vi "NI-DAQmxUpdate.vi"() -> (0 "error out":errorcluster)   [LabVIEW 2022 SP3]
uses:
  Sub_vis/Upload Data.ctl
  <vilib>/DAQmx/read.llb/DAQmx Read (Analog 2D DBL NChan NSamp).vi
  Globals/Meas_global.vi
  <vilib>/DAQmx/create/channels.llb/DAQmx Create Channel (AI-Voltage-Basic).vi
  PWA/PWAtasksGLOBAL.vi
  <vilib>/DAQmx/configure/timing.llb/DAQmx Timing (Sample Clock).vi
  <vilib>/DAQmx/miscellaneous.llb/DAQmx Fill In Error Info.vi
  <resource>/objmgr/daqmx.rc
  5b8cb71c-e545-4ba2-a204-efceee465973.vi
panel:
  out "bufferSizeAssigned":u32
  out "totalPlannedSamples":i32
  out "Array":string[](array[string])
  out "Requested No of blocks":i32
  out "Current Block No":i32
  out "FsReq":dbl
  out "FsRead":dbl format="%#_11g"
  out "input terminal configuration":i32(ring)=10106 items=["default"=-1, "RSE"=10083, "NRSE"=10078, "Differential"=10106, "Pseudodifferential"=12529]
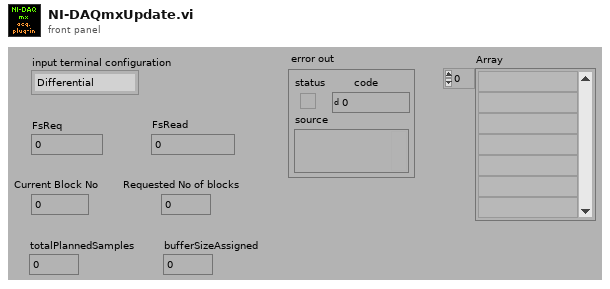
[diagram p1: front panel]
types:
  T1 = typedef "Analysis_info_cluster.ctl" = cluster{"Colour":u32, "Inst type":T2, "Inst name":string, "Symbol":string, "Code name":string, "Extra Info":string, "Inst Array":T3, "U":dbl, "u^2":dbl, "u^3":dbl, "u^4":dbl, "Skew_u":dbl, "Kurt_u":dbl, "Sd Error in Mean":dbl, "% u'/U":dbl, "X":dbl, "Y":dbl, "Z":dbl, "Timescale integral Estimate":dbl, "Sd Error in Variance":dbl, "Calib File":path, "Calib Constants":dbl[], "Output Position":bool, "Stats":enum16{"None", "Basic", "Full"}, "Av Sampling Rate":dbl, "Av No of Samples":dbl, "Total Meas Time (s)":dbl, "OrigChName":string, "Max value":dbl, "Min value":dbl, "Req Sample Rate Hz":dbl, "Sync Delay Time (s)":dbl, "Ch No":i16, "Device":string, "Use Latest Calib":bool, "Port":string, "Metadata Ch Names":string[], "Metadata Ch Values":string[], "Label":string, "chState":T4, "Point Drift":dbl, "inputConfig":string}
  T2 = typedef "Inst_type.ctl" = enum16{"Raw voltage", "Raw with zero offsetting", "Propeller anemometer", "Pressure Transducer", "Pitot-static tube", "Hot wire", "Cross wire 1", "Cross wire 2", "Generic Linear", "Generic Polynomial", "Generic BackPoly", "Fast FID", "Thermocouple", "Cold wire", "Pulsed Wire", "LDA Vel", "LDA Tran time", "LDA Arr time", "Microphone"}
  T3 = typedef "Instrument_Array.ctl" = enum16{"PWA", "LDA", "Analogue"}
  T4 = typedef "channelState.ctl" = enum32{"No Selection", "Solo", "Mute"}
  T5 = typedef "Device ID port info.ctl" = cluster{"Ch No":i16[], "Req Sampling Rate":dbl[], "Port":string, "Index":i32[]}
  T6 = typedef "Upload Data.ctl" = enum16{"Voltage Array", "Time Trace Cluster"}
  T7 = typedef "Setup.ctl" = enum16{"Run Program", "Show Setup", "Save Current Setup", "Setup Front Panel"}
  T8 = typedef "Rendezvous RefNum" = refnum<k1>
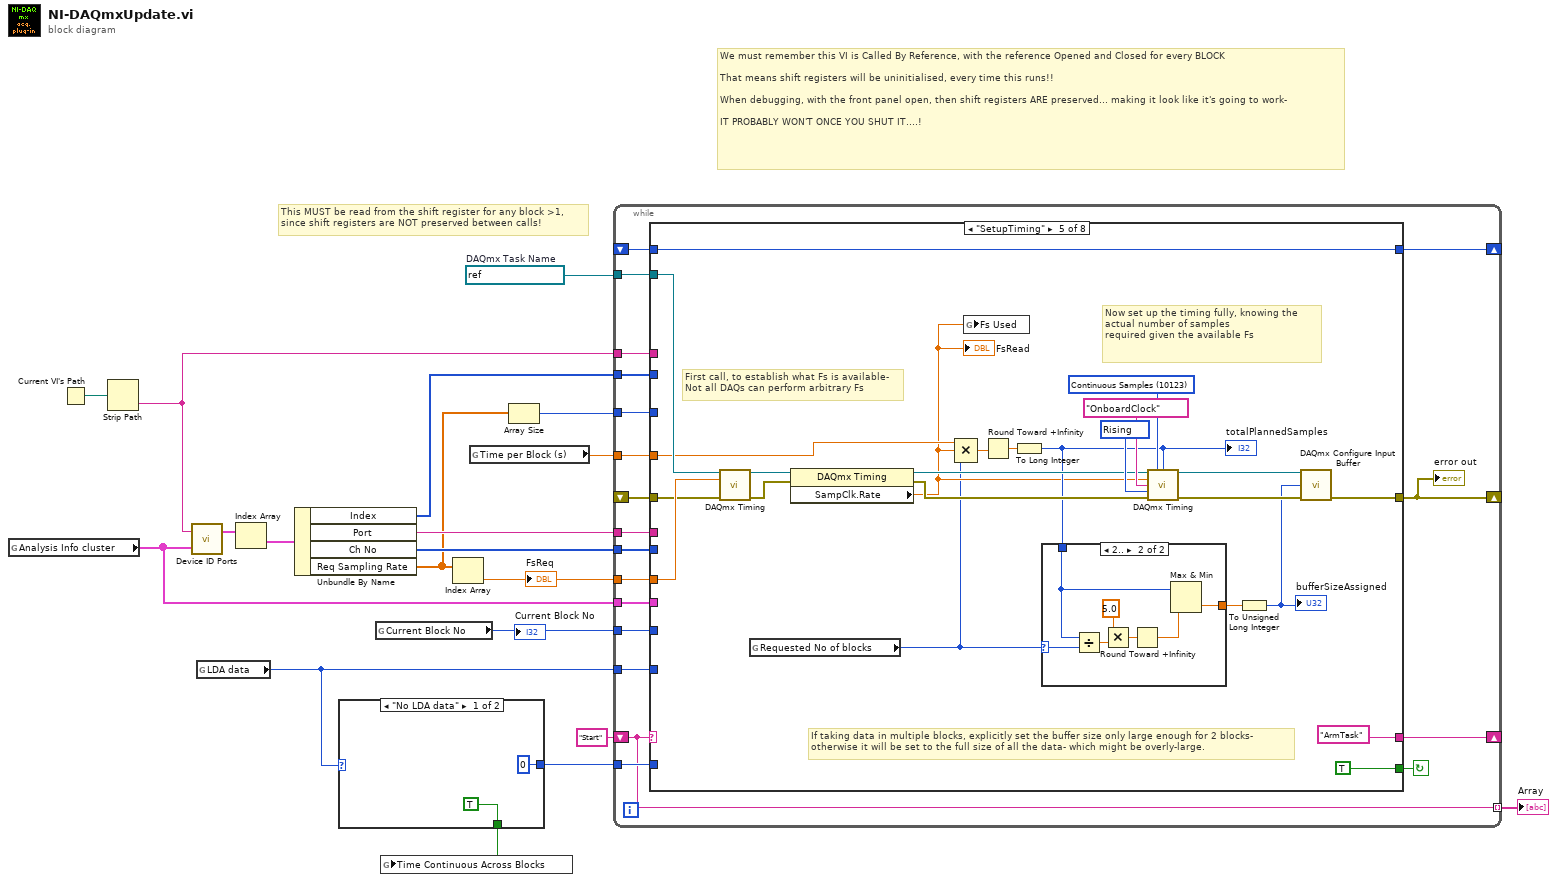
[diagram p0: block diagram]
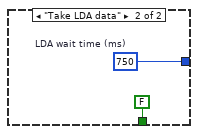
[diagram p2: hidden frame]
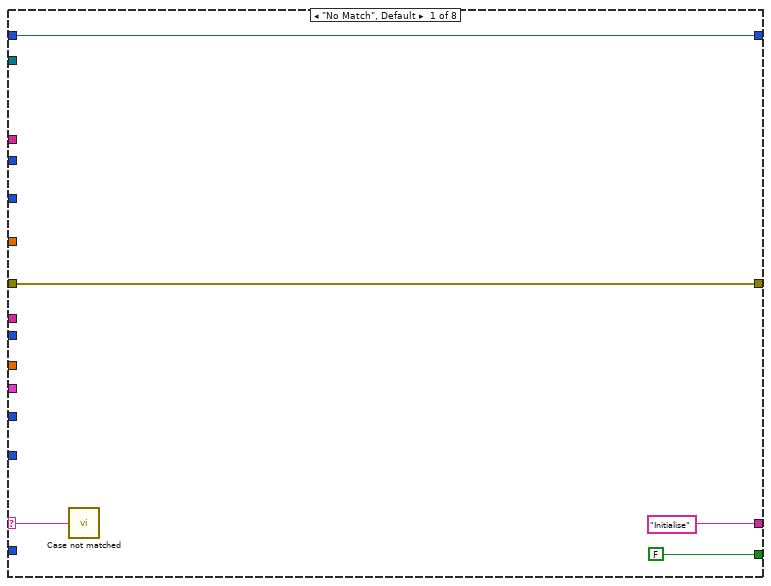
[diagram p3: hidden frame]
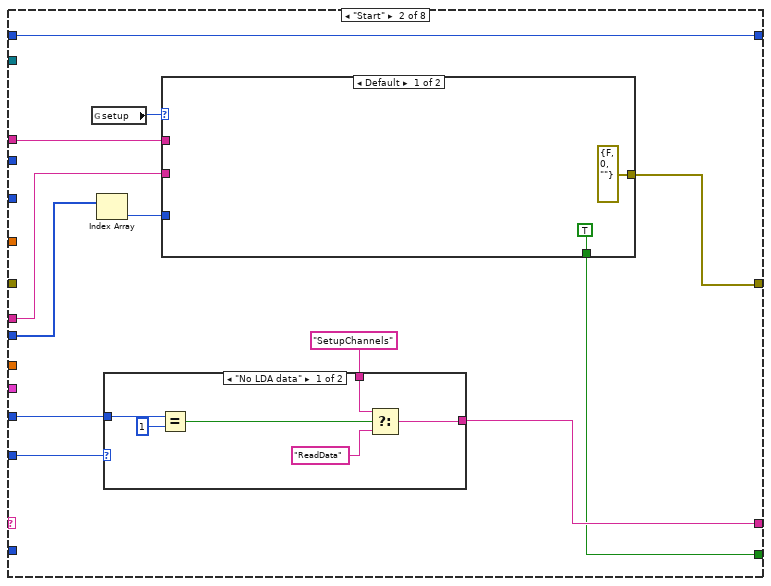
[diagram p4: hidden frame]
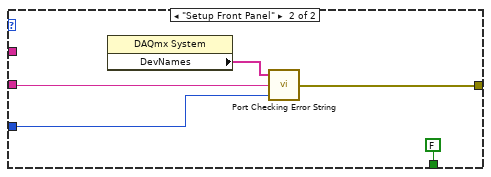
[diagram p5: hidden frame]
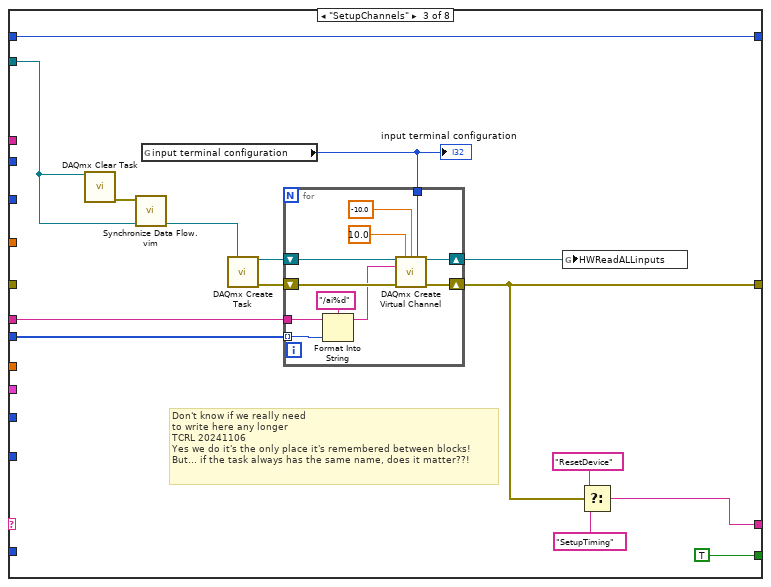
[diagram p7: hidden frame]
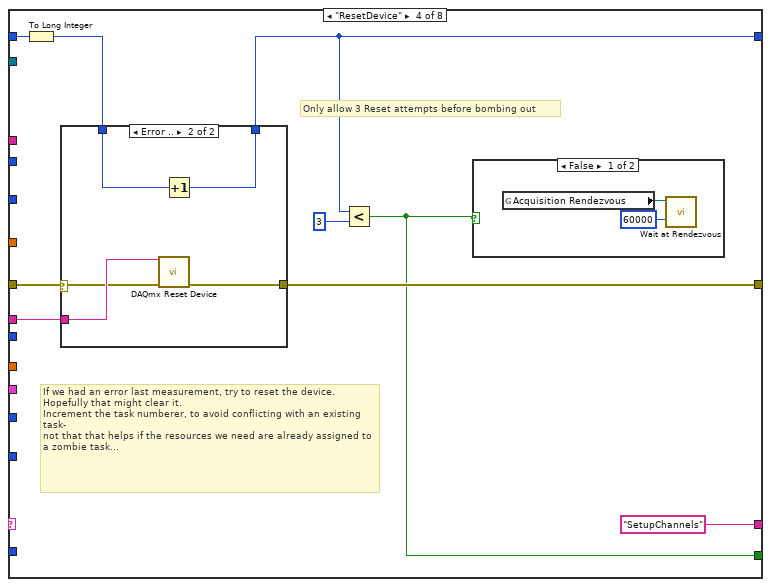
[diagram p8: hidden frame]
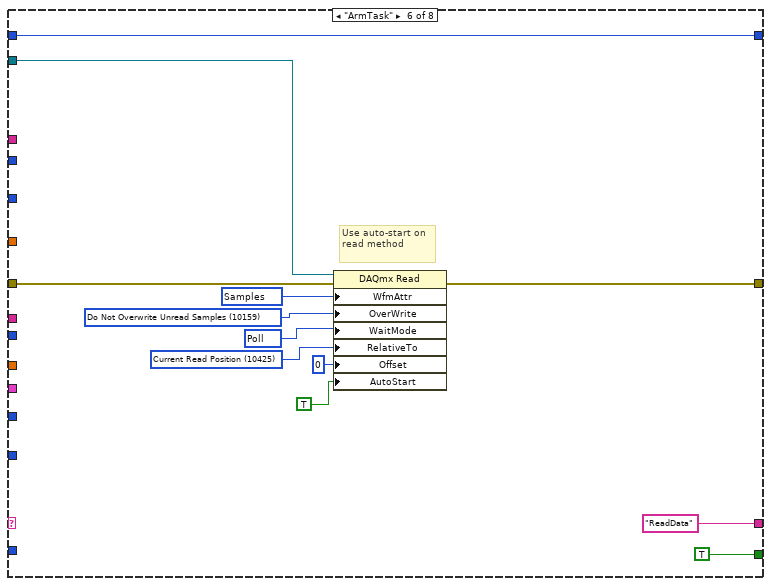
[diagram p12: hidden frame]
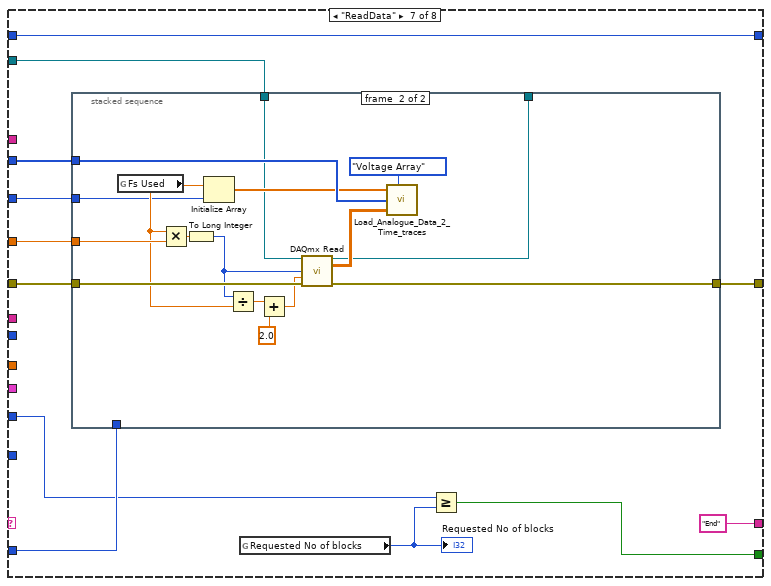
[diagram p13: hidden frame]
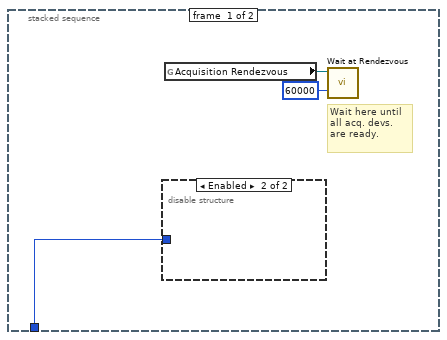
[diagram p14: hidden frame]
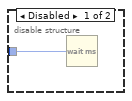
[diagram p15: hidden frame]
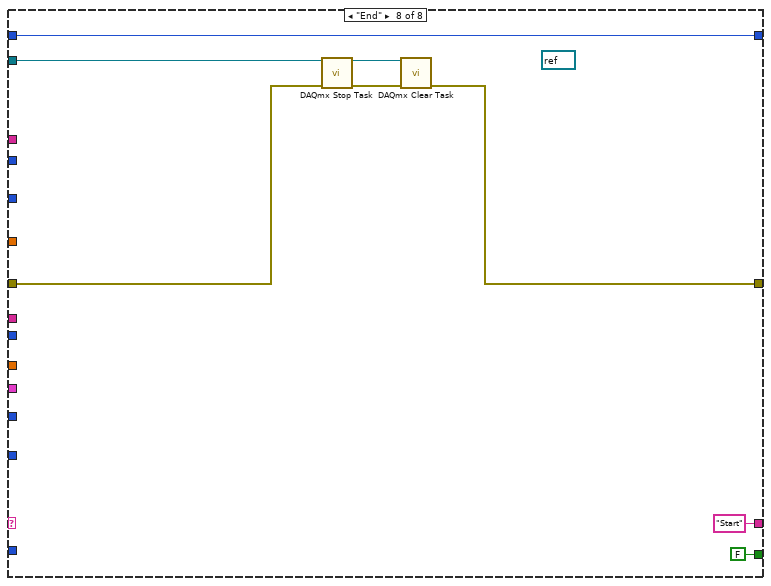
[diagram p16: hidden frame]
diagram:
  w1 = refnum<k21> "EnFloDAQmx"  # DAQmx Task Name
  # "This MUST be read from the shift register for any block >1,\nsince shift registers are NOT preserved between calls!"
  # "We must remember this VI is Called By Reference, with the reference Opened and Closed for every BLOCK\n\nThat means shift registers will be uninitialised, every time this runs!!\n\nWhen debugging, with the front panel open, then shift registers ARE preserved... making it look like it's going to work-\n\nIT PROBABLY WON'T ONCE YOU SHUT IT....!"
  n1 = global read "Meas_global.vi" "Analysis Info cluster"() -> (w8:T1[])
  n2 = Current VI's Path() -> (path=w15:path)
  n3 = Strip Path(path=w15) -> (name=w9:string)  [unwired: 1 out]
  n4 = call "Device ID Ports.vi"("Analysis Info cluster"=w8, "DAQdeviceType"=w9) -> ("Device port info"=w14:T5[])  [unwired: 1 out]
  n5 = global read "Meas_global.vi" "LDA data"() -> (w18:enum16{"No LDA data", "Take LDA data"})
  n6 = Index Array(array=w14) -> (element=w13:T5)  [unwired: 1 in]
  n7 = Unbundle By Name(w13) -> ("Index"=w11:i32[], "Port"=w12:string, "Ch No"=w10:i16[], "Req Sampling Rate"=w4:dbl[])
  n8 = case shown="\"No LDA data\"" w18 {
    tunnel: [TRUE ("Time Continuous across Blocks") FALSE ("Time Continuous across Blocks")] -> w17
    tunnel: [u32 0 ("LDA wait time (ms)") w22] -> w16
    frame "No LDA data" {
    }
    frame "Take LDA data" {
      w22 = u32 750  # LDA wait time (ms)
    }
  }
  n9 = global read "Meas_global.vi" "Current Block No"() -> (w6:i32)
  "Current Block No" <- w6
  n10 = global write "Meas_global.vi" "Time Continuous Across Blocks"(w17) -> ()
  n11 = Index Array(array=w4) -> (element=w3:dbl)  [unwired: 1 in]
  "FsReq" <- w3
  n12 = global read "Meas_global.vi" "Time per Block (s)"() -> (w7:dbl)
  n13 = Array Size(array=w4) -> (size(s)=w5:i32)
  n14 = while {
    shift-left: "Start" -> [w24]
    shift-right: [w25] -> _
    shift-right: [w27] -> _
    shift-left: _ -> [w26]
    tunnel: w3 -> [w42]
    tunnel: w6 -> [w41]
    shift-right: [w40] -> _
    shift-left: _ -> [w39]
    tunnel: w18 -> [w38]
    tunnel: w16 -> [w37]
    tunnel: w10 -> [w36]
    tunnel: w12 -> [w35]
    tunnel: w11 -> [w34]
    tunnel: w9 -> [w33]
    tunnel: w8 -> [w32]
    tunnel: w7 -> [w30]
    tunnel: w5 -> [w28]
    tunnel: [w24] -> w2 mode=indexing
    tunnel: w1 -> [w29]
    stop <- w31 continue-if-true
    n15 = case shown="\"SetupTiming\"" w24 {
      selector: w24 -> [w43 _ _ _ _ _ _ _]
      tunnel: [FALSE w48 TRUE w100 TRUE TRUE w165 FALSE] -> w31
      tunnel: ["Initialise" w58 w78 "SetupChannels" "ArmTask" "ReadData" "End" "Start" ("f")] -> w25
      tunnel: [w45 w49 w80 w105 w124 w157 w168 w198] -> w27
      tunnel: w26 -> [w45 _ _ w103 w136 w160 w173 w195]
      tunnel: w42 -> [_ _ _ _ w138 _ _ _]
      tunnel: w41 -> [_ w56 _ _ _ _ w164 _]
      tunnel: [w44 w57 w85 w102 w139 w158 w171 w199] -> w40
      tunnel: w39 -> [w44 w57 w85 w107 w139 w158 w171 w199]
      tunnel: w38 -> [_ w55 _ _ _ _ _ _]
      tunnel: w37 -> [_ _ _ _ _ _ w170 _]
      tunnel: w36 -> [_ w51 w84 _ _ _ _ _]
      tunnel: w35 -> [_ w52 w83 w106 _ _ _ _]
      tunnel: w34 -> [_ _ _ _ _ _ w169 _]
      tunnel: w33 -> [_ w54 _ _ _ _ _ _]
      tunnel: w32 -> [_ _ _ _ _ _ _ _]
      tunnel: w30 -> [_ _ _ _ w121 _ w167 _]
      tunnel: w29 -> [_ _ w75 _ w137 w156 w162 w194]
      tunnel: w28 -> [_ _ _ _ _ _ w166 _]
      frame "No Match", Default {
        n16 = call "Case not matched.vi"("Case Name not Matched"=w43) -> ()
      }
      frame "Start" {
        n17 = global read "Meas_global.vi" "setup"() -> (w53:T7)
        n18 = Index Array(array=w51) -> (element=w50:i16)  [unwired: 1 in]
        n19 = case shown="\"No LDA data\"" w55 {
          tunnel: "SetupChannels" -> [w72 w73]
          tunnel: [w70 w73] -> w58
          tunnel: w56 -> [w69 _]
          frame "No LDA data" {
            n20 = Equal?(x=w69, y=1) -> (x = y?=w67:bool)
            n21 = Select(t=w72, s=w67, f="ReadData") -> (s? t:f=w70:string)
          }
          frame "Take LDA data" {
          }
        }
        n22 = case shown="Default" w53 {
          tunnel: w54 -> [_ _]
          tunnel: w52 -> [_ w65]
          tunnel: w50 -> [_ w66]
          tunnel: [errorcluster {"status"=FALSE, "code"=0, "source"=""} ("error out") w64] -> w49
          tunnel: [TRUE FALSE] -> w48
          frame Default {
          }
          frame "Setup Front Panel" {
            n23 = property class="DAQmx System"() -> ("DevNames"=w62:tag[])  [unwired: 2 in, 2 out]
            n24 = call "Port Checking Error String.vi"("Ch Index"=w66, "Port"=w65, "Available Ports"=w62) -> ("error out"=w64:errorcluster)  [unwired: 1 in]
          }
        }
      }
      frame "SetupChannels" {
        # "Don't know if we really need\nto write here any longer\nTCRL 20241106\nYes we do it's the only place it's remembered between blocks!\nBut... if the task always has the same name, does it matter??!"
        n25 = call <vilib>:"DAQmx Clear Task.vi"("task in"=w75) -> ("error out"=w76:errorcluster)  [unwired: 14 in]
        n26 = call "Synchronize Data Flow.vim"("input 4"=w75, "input 1"=w76) -> ("output 4"=w74:refnum<k21>)  [unwired: 2 in, 3 out]
        n27 = global read "Meas_global.vi" "input terminal configuration"() -> (w81:i32)
        "input terminal configuration" <- w81
        n28 = call <vilib>:"DAQmx Create Task.vi"("new task name"=w74) -> ("task out"=w87:refnum<k21>, "error out"=w88:errorcluster)  [unwired: 4 in, 9 out]
        n29 = for {
          shift-right: [w98] -> w82
          shift-left: w87 -> [w99]
          shift-right: [w96] -> w80
          shift-left: w88 -> [w97]
          tunnel: w84 -> [w93] mode=indexing
          tunnel: w83 -> [w92]
          tunnel: w81 -> [w89]
          n30 = Format Into String(format string="/ai%d", initial string=w92, w93) -> (resulting string=w94:string)  [unwired: 1 in, 1 out]
          n31 = call-poly <vilib>:"DAQmx Create Virtual Channel.vi"("task in"=w99, "maximum value"=10.0, "minimum value"=-10.0, "input terminal configuration"=w89, "physical channels"=w94, "error in"=w97) -> ("task out"=w98:refnum<k21>, "error out"=w96:errorcluster)  [unwired: 3 in, 5 out]
        }
        n32 = global write "PWAtasksGLOBAL.vi" "HWReadALLinputs"(w82) -> ()
        n33 = Select(t="ResetDevice", s=w80, f="SetupTiming") -> (s? t:f=w78:string)
      }
      frame "ResetDevice" {
        # "Only allow 3 Reset attempts before bombing out"
        # "If we had an error last measurement, try to reset the device.\nHopefully that might clear it.\nIncrement the task numberer, to avoid conflicting with an existing task-\nnot that that helps if the resources we need are already assigned to a zombie task..."
        n34 = To Long Integer(number=w107) -> (32bit integer=w104:i32)
        n35 = case shown="Error .." w103 {
          selector: w103 -> [w112 w113]
          tunnel: w106 -> [_ w117]
          tunnel: [w112 w114] -> w105
          tunnel: w104 -> [w111 w116]
          tunnel: [w111 w115] -> w102
          frame No Error {
          }
          frame Error {
            n36 = call <vilib>:"DAQmx Reset Device.vi"("device in"=w117, "error in"=w113) -> ("error out"=w114:errorcluster)  [unwired: 13 in]
            n37 = Increment(x=w116) -> (x+1=w115:i32)
          }
        }
        n38 = Less?(x=w102, y=3) -> (x < y?=w100:bool)
        n39 = case shown="False" w100 {
          frame False {
            n40 = global read "Meas_global.vi" "Acquisition Rendezvous"() -> (w110:T8)
            n41 = call <vilib>:"Wait at Rendezvous.vi"("ms timeout (-1)"=60000, "rendezvous"=w110) -> ()  [unwired: 3 in, 3 out]
          }
          frame True {
          }
        }
      }
      frame "SetupTiming" {
        w132 = 10280 items=["Rising"=10280, "Falling"=10171] ("active edge")
        w134 = 10123 items=["Finite Samples"=10178, "Continuous Samples"=10123, "Hardware Timed Single Point"=12522] ("sample mode")
        # "If taking data in multiple blocks, explicitly set the buffer size only large enough for 2 blocks-\notherwise it will be set to the full size of all the data- which might be overly-large."
        # "Now set up the timing fully, knowing the actual number of samples\nrequired given the available Fs"
        # "First call, to establish what Fs is available-\nNot all DAQs can perform arbitrary Fs"
        n42 = call-poly <vilib>:"DAQmx Timing.vi"("task/channels in"=w137, "rate"=w138, "error in"=w136) -> ("task out"=w135:refnum<k21>, "error out"=w130:errorcluster)  [unwired: 4 in, 7 out]
        n43 = global read "Meas_global.vi" "Requested No of blocks"() -> (w118:i32)
        n44 = property class="DAQmx Timing"(reference=w135, error in=w130) -> (reference out=w131:refnum<k21>, error out=w129:errorcluster, "SampClk.Rate"=w120:dbl)
        "FsRead" <- w120
        n45 = Compound Arithmetic op=MULTIPLY(w121, w120, w118) -> (w119:dbl)
        n46 = global write "Meas_global.vi" "Fs Used"(w120) -> ()
        n47 = Round Toward +Infinity(x=w119) -> (ceil(x): smallest int >= x=w128:dbl)
        n48 = To Long Integer(number=w128) -> (32bit integer=w127:i32)
        "totalPlannedSamples" <- w127
        n49 = case shown="2.." w118 {
          selector: w118 -> [_ w147]
          tunnel: w127 -> [w142 w145]
          tunnel: [w142 w143] -> w123
          frame 1, Default {
          }
          frame 2.. {
            n50 = Divide(x=w145, y=w147) -> (x/y=w149:dbl)
            n51 = Multiply(x=5.0, y=w149) -> (x*y=w146:dbl)
            n52 = Round Toward +Infinity(x=w146) -> (ceil(x): smallest int >= x=w144:dbl)
            n53 = Max & Min(x=w145, y=w144) -> (min(x,y)=w143:dbl)  [unwired: 1 out]
          }
        }
        n54 = call-poly <vilib>:"DAQmx Timing.vi"("task/channels in"=w131, "sample mode"=w134, "samples per channel"=w127, "rate"=w120, "source"=tag "OnboardClock", "active edge"=w132, "error in"=w129) -> ("task out"=w125:refnum<k21>, "error out"=w126:errorcluster)  [unwired: 7 out]
        n55 = To Unsigned Long Integer(number=w123) -> (unsigned 32bit integer=w122:u32)
        "bufferSizeAssigned" <- w122
        n56 = call <vilib>:"DAQmx Configure Input Buffer.vi"("task/channels in"=w125, "buffer size (in samples per channel)"=w122, "error in"=w126) -> ("error out"=w124:errorcluster)  [unwired: 11 in, 1 out]
      }
      frame "ArmTask" {
        w152 = 10425 items=["First Sample"=10424, "Current Read Position"=10425, "Reference Trigger"=10426, "First Pretrigger Sample"=10427, "Most Recent Sample"=10428] ("RelativeTo")
        w153 = 12524 items=["Wait For Interrupt"=12523, "Poll"=12524, "Yield"=12525, "Sleep"=12547] ("WaitMode")
        w154 = 10159 items=["Overwrite Unread Samples"=10252, "Do Not Overwrite Unread Samples"=10159] ("OverWrite")
        w155 = 10287 items=["Samples"=10287, "Samples and Timing"=10140, "Samples, Timing, and Attributes"=10141] ("WfmAttr")
        # "Use auto-start on read method"
        n57 = property class="DAQmx Read"(reference=w156, error in=w160, "WfmAttr"=w155, "OverWrite"=w154, "WaitMode"=w153, "RelativeTo"=w152, "Offset"=0, "AutoStart"=TRUE) -> (error out=w157:errorcluster)  [unwired: 1 out]
      }
      frame "ReadData" {
        n58 = stacked-sequence {
          tunnel: w173 -> [_ w193]
          tunnel: [_ w192] -> w168
          tunnel: w170 -> [w176 _]
          tunnel: w169 -> [_ w187]
          tunnel: w167 -> [_ w183]
          tunnel: w166 -> [_ w180]
          tunnel: [_ w179] -> _
          tunnel: w162 -> [_ w178]
          frame #0 {
            # "Wait here until all acq. devs. are ready."
            n59 = disable-structure shown="Enabled" {
              disable-tunnel: w176 -> [w177 _]
              frame Disabled {
                n60 = Wait (ms)(milliseconds to wait=w177) -> ()  [unwired: 1 out]
              }
              frame Enabled {
              }
            }
            n61 = global read "Meas_global.vi" "Acquisition Rendezvous"() -> (w175:T8)
            n62 = call <vilib>:"Wait at Rendezvous.vi"("ms timeout (-1)"=60000, "rendezvous"=w175) -> ()  [unwired: 3 in, 3 out]
          }
          frame #1 {
            n63 = global read "Meas_global.vi" "Fs Used"() -> (w182:dbl)
            n64 = Multiply(x=w182, y=w183) -> (x*y=w184:dbl)
            n65 = To Long Integer(number=w184) -> (32bit integer=w181:i32)
            n66 = Initialize Array(w182, w180) -> (w186:dbl[])
            n67 = Divide(x=w181, y=w182) -> (x/y=w191:dbl)
            n68 = Add(x=w191, y=2.0) -> (x+y=w189:dbl)
            n69 = call-poly <vilib>:"DAQmx Read.vi"("task/channels in"=w178, "number of samples per channel"=w181, "timeout"=w189, "error in"=w193) -> ("task out"=w179:refnum<k21>, "data"=w188:dbl[][], "error out"=w192:errorcluster)  [unwired: 9 out]
            n70 = call "Load_Analogue_Data_2_Time_traces.vi"("Sampling Rate (Hz)"=w186, "Mode"=Upload_Data."Voltage Array", "Index"=w187, "Voltage Array"=w188) -> ()  [unwired: 3 in]
          }
        }
        n71 = global read "Meas_global.vi" "Requested No of blocks"() -> (w163:i32)
        "Requested No of blocks" <- w163
        n72 = Greater Or Equal?(x=w164, y=w163) -> (x >= y?=w165:bool)
      }
      frame "End" {
        (unwired) refnum<k21> refnum ("task out")
        n73 = call <vilib>:"DAQmx Stop Task.vi"("task/channels in"=w194, "error in"=w195) -> ("task out"=w197:refnum<k21>, "error out"=w196:errorcluster)  [unwired: 12 in]
        n74 = call <vilib>:"DAQmx Clear Task.vi"("task in"=w197, "error in"=w196) -> ("error out"=w198:errorcluster)  [unwired: 13 out]
      }
    }
    "error out" <- w27
  }
  "Array" <- w2
